vi "Configure Waveform (Noise).vi"(0 "VISA resource name":refnum<visa-resource-name>, 9 "Amplitude (1.0 Vpp)":dbl=1.0, 11 "error in (no error)":errorcluster, 12 "DC Offset (0.00 V)":dbl) -> (4 "VISA resource name out":refnum<visa-resource-name>, 15 "error out":errorcluster)   [LabVIEW 2017, in "Keithley 3390.lvlib"]
doc: "Sets the waveform parameters for a noise waveform and makes it the active waveform function."
uses:
  Keithley 3390.lvlib
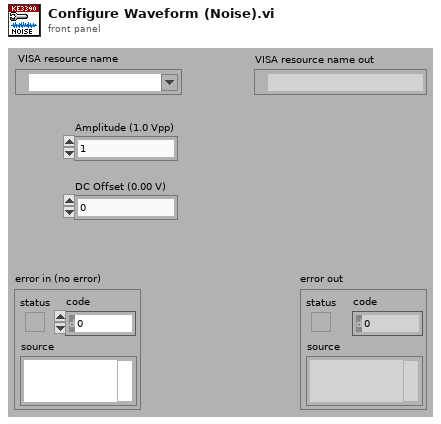
[diagram p1: front panel]
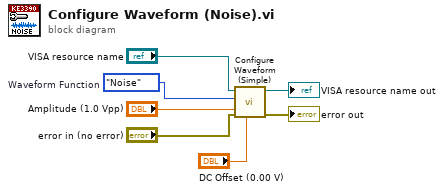
[diagram p0: block diagram]
diagram:
  w1 = enum16{"Sine", "Noise", "DC"}."Noise"  # Waveform Function
  n1 = call "Configure Waveform (Simple).vi"("DC Offset (0.00 V)"="DC Offset (0.00 V)", "error in (no error)"="error in (no error)", "Amplitude (1.0 Vpp)"="Amplitude (1.0 Vpp)", "Waveform Function (0: Sine)"=w1, "VISA resource name"="VISA resource name") -> ("error out"=→"error out":errorcluster, "VISA resource name out"=→"VISA resource name out":refnum<visa-resource-name>)  [unwired: 5 in]
